vi "CTRE_Phoenix_CANdle_SetControlFramePeriod.vi"(8 "error in (no error)":errorcluster, 9 "periodMs":i32, 10 "CANdle Control Frame":T1=262144 items=["Control_1_General"=262144, "Control_2_ModulatedVBatOutput"=262208], 11 "CTRE_CANdle_DeviceRef":T2) -> (0 "error out":errorcluster, 3 "CTRE_CANdle_DeviceRef":T2)   [LabVIEW 2020]
doc: "Set the period of the specified control frame."
uses:
  <vilib>/Rock Robotics/WPI/ThirdParty/Phoenix-LabVIEW/CANdle/Controls/CTRE_Phoenix_CANdle_DeviceRef.ctl
  <vilib>/Rock Robotics/WPI/ThirdParty/Phoenix-LabVIEW/CANdle/Controls/CTRE_Phoenix_CANdle_ControlFrame.ctl
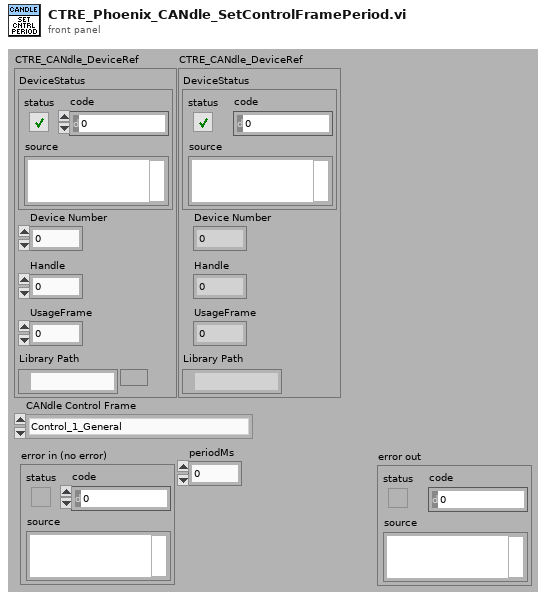
[diagram p1: front panel]
types:
  T1 = typedef "CTRE_Phoenix_CANdle_ControlFrame.ctl" = u32
  T2 = typedef "CTRE_Phoenix_CANdle_DeviceRef.ctl" = cluster{"DeviceStatus":errorcluster, "Device Number":u8, "Handle":u64, "UsageFrame":u32, "Library Path":path}
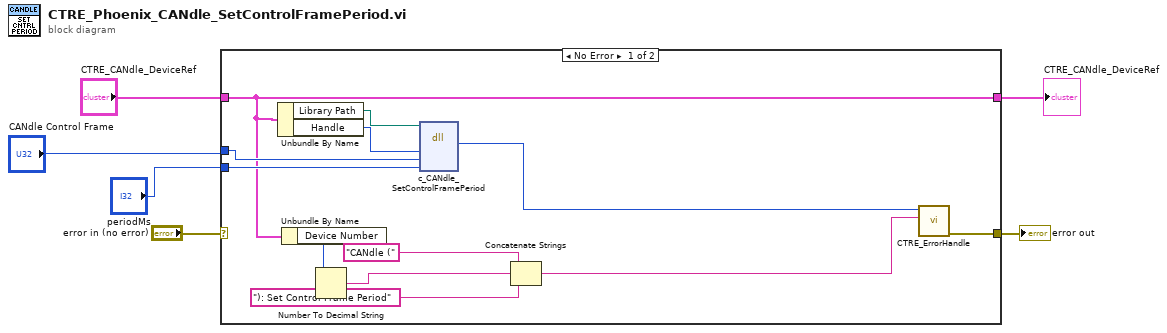
[diagram p0: block diagram]
diagram:
  n1 = case shown="No Error" "error in (no error)" {
    selector: "error in (no error)" -> [_ w20]
    tunnel: [w14 w20] -> w6
    tunnel: "CTRE_CANdle_DeviceRef" -> [w9 w19]
    tunnel: [w9 w19] -> w2
    tunnel: "CANdle Control Frame" -> [w11 _]
    tunnel: "periodMs" -> [w10 _]
    frame No Error {
      n2 = Unbundle By Name(w9) -> ("Library Path"=w8:path, "Handle"=w7:u64)
      n3 = Unbundle By Name(w9) -> ("Device Number"=w15:u8)
      n4 = Number To Decimal String(number=w15) -> (decimal integer string=w17:string)  [unwired: 1 in]
      n5 = dll-call lib="?" fn="c_CANdle_SetControlFramePeriod"(path in=w8, "handle"=w7, "frame"=w11, "periodMs"=w10) -> ("ErrorCode"=w12:i32)  [unwired: 5 in, 2 out]
      n6 = Concatenate Strings("CANdle (" ("string"), w17, "): Set Control Frame Period" ("string")) -> (w13:string)
      n7 = call <vilib>:"CTRE_ErrorHandle.vi"("origin"=w13, "code"=w12) -> ("error out"=w14:errorcluster)  [unwired: 9 in]
    }
    frame Error {
    }
  }
  "error out" <- w6
  "CTRE_CANdle_DeviceRef" <- w2
